vi "Vision Main.vi"(10 "Cropped Image":T1, 11 "Camera Image":T1(plugin-control)) -> (2 "Chosen Target Angle":dbl, 3 "Sorted Targets":T2(array[cluster]))   [LabVIEW 2012]
uses:
  <vilib>/vision/Image Controls.llb/IMAQ Image.ctl
panel:
  out "Particle Reports (Pixels)":T3(array[cluster]) {"Orientation" format="%.2f"; "Dimensions"."Height" format="%.2f"; "Dimensions"."Width" format="%.2f"; "Center of Mass"."Y" format="%.2f"; "Center of Mass"."X" format="%.2f"; "Bounding Rect"."Bottom" format="%.2f"; "Bounding Rect"."Right" format="%.2f"; "Bounding Rect"."Top" format="%.2f"; "Bounding Rect"."Left" format="%.2f"; "Number of Holes" format="%.2f"; "Area" format="%.2f"}
  out "Number of Particles":i32
  out "Processed Image":T1(plugin-control)
  out "Cropped Image":T1(plugin-control)
  # "Camera Image"
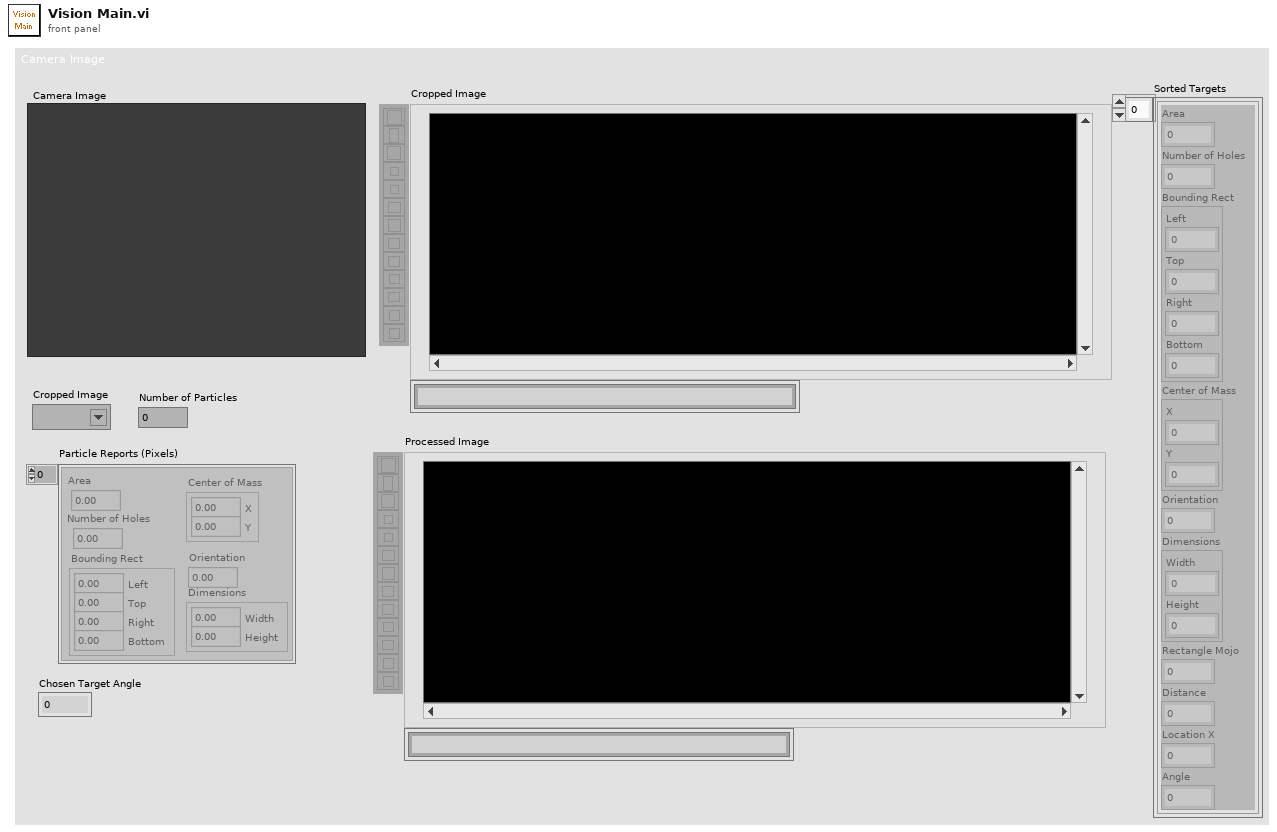
[diagram p1: front panel]
types:
  T1 = typedef "IMAQ Image.ctl" = refnum<image>
  T2 = cluster{"Area":dbl, "Number of Holes":dbl, "Bounding Rect":cluster{"Left":dbl, "Top":dbl, "Right":dbl, "Bottom":dbl}, "Center of Mass":cluster{"X":dbl, "Y":dbl}, "Orientation":dbl, "Dimensions":cluster{"Width":dbl, "Height":dbl}, "Rectangle Mojo":dbl, "Distance":dbl, "Location X":dbl, "Angle":dbl}[]
  T3 = cluster{"Area":dbl, "Number of Holes":dbl, "Bounding Rect":cluster{"Left":dbl, "Top":dbl, "Right":dbl, "Bottom":dbl}, "Center of Mass":cluster{"X":dbl, "Y":dbl}, "Orientation":dbl, "Dimensions":cluster{"Width":dbl, "Height":dbl}}[]
  T4 = typedef "Image Type" = u32
  T5 = cluster{"Area":dbl, "Number of Holes":dbl, "Bounding Rect":cluster{"Left":dbl, "Top":dbl, "Right":dbl, "Bottom":dbl}, "Center of Mass":cluster{"X":dbl, "Y":dbl}, "Orientation":dbl, "Dimensions":cluster{"Width":dbl, "Height":dbl}, "Rectangle Mojo":dbl, "Distance":dbl, "Location X":dbl, "Angle":dbl}
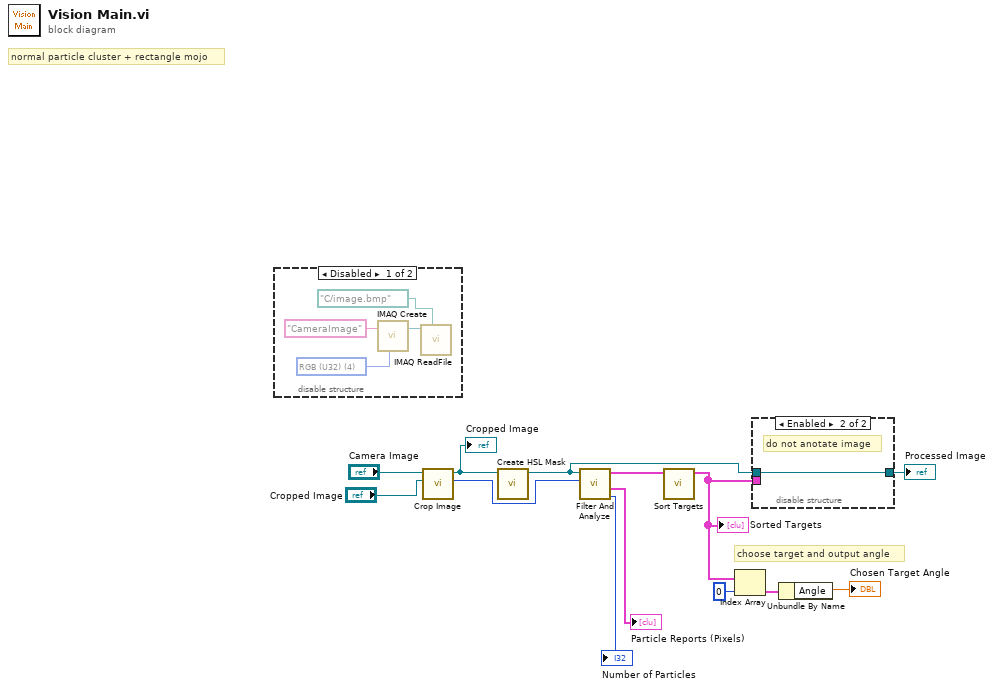
[diagram p0: block diagram]
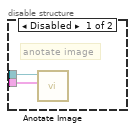
[diagram p2: hidden frame]
diagram:
  # "choose target and output angle"
  # "normal particle cluster + rectangle mojo"
  n1 = disable-structure shown="Disabled" {
    frame Disabled {
      w15 = T4 4 items=["Grayscale (U8)", "Grayscale (I16)", "Grayscale (SGL)", "Complex (CSG)", "RGB (U32)", "HSL (U32)", "RGB (U64)", "Grayscale (U16)"] ("Image Type")
      n2 = call "IMAQ Create"("Image Name"="CameraImage", "Image Type"=w15) -> ("New Image"=w18:T1)  [unwired: 3 in, 1 out]
      n3 = call "IMAQ ReadFile"("File Path"=path "C:/image.bmp", "Image"=w18) -> ("Image Out"=w14:T1)  [unwired: 5 in, 4 out]
    }
    frame Enabled {
    }
  }
  n4 = call "Crop Image.vi"("Cropped Image"="Cropped Image", "Camera Image"="Camera Image") -> ("Y Resolution"=w10:i32, "Cropped Image"=w12:T1)  [unwired: 7 in, 1 out]
  "Cropped Image" <- w12
  n5 = call "Create HSL Mask.vi"("Cropped Image"=w12) -> ("Image Mask"=w11:T1)  [unwired: 10 in]
  n6 = call "Filter And Analyze.vi"("Y Resolution"=w10, "Refnum in"=w11) -> ("Number of Particles"=→"Number of Particles":i32, "Particle Reports (Pixels)"=→"Particle Reports (Pixels)":T3, "Filtered Array"=w9:T2)  [unwired: 7 in]
  n7 = call "Sort Targets.vi"("Filtered Array"=w9) -> ("Sorted Array"=w6:T2)  [unwired: 10 in]
  "Sorted Targets" <- w6
  n8 = Index Array(array=w6, index=0) -> (element=w4:T5)
  n9 = disable-structure shown="Enabled" {
    disable-tunnel: w11 -> [w21 w22]
    disable-tunnel: w6 -> [w20 _]
    disable-tunnel: [_ w22] -> w2
    frame Disabled {
      # "anotate image"
      n10 = call "Anotate Image.vi"("Sorted Array"=w20, "Image Refnum in"=w21) -> ("Image Refnum out"=w19:T1)  [unwired: 9 in]
    }
    frame Enabled {
      # "do not anotate image"
    }
  }
  "Processed Image" <- w2
  n11 = Unbundle By Name(w4) -> ("Angle"=→"Chosen Target Angle":dbl)
